vi "WiseDrive.vi"(8 "error in":errorcluster, 11 "Joystick Input":dbl(slide) scale=-1.0..1.0) -> (0 "error out":errorcluster, 3 "Throttle":dbl)   [LabVIEW 2015]
panel:
  in  "Low slope":dbl=0.5
  in  "Switch value":dbl=0.7
  # "remember to set as default to configure"
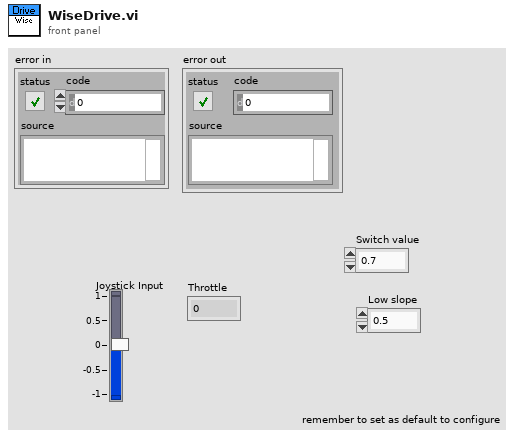
[diagram p1: front panel]
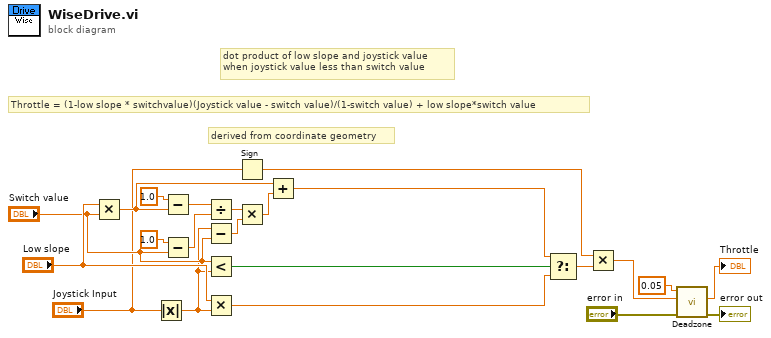
[diagram p0: block diagram]
diagram:
  # "derived from coordinate geometry"
  # "Throttle = (1-low slope * switchvalue)(Joystick value - switch value)/(1-switch value) + low slope*switch value"
  # "dot product of low slope and joystick value \nwhen joystick value less than switch value"
  n1 = Multiply(x="Low slope", y="Switch value") -> (x*y=w14:dbl)
  n2 = Absolute Value(x="Joystick Input") -> (abs(x)=w5:dbl)
  n3 = Subtract(x=1.0, y=w14) -> (x-y=w13:dbl)
  n4 = Subtract(x=1.0, y="Switch value") -> (x-y=w11:dbl)
  n5 = Divide(x=w13, y=w11) -> (x/y=w10:dbl)
  n6 = Subtract(x=w5, y="Switch value") -> (x-y=w9:dbl)
  n7 = Less?(x="Switch value", y=w5) -> (x < y?=w17:bool)
  n8 = Multiply(x="Low slope", y=w5) -> (x*y=w18:dbl)
  n9 = Sign(1:"Joystick Input") -> (0:w3:dbl)
  n10 = Multiply(x=w10, y=w9) -> (x*y=w8:dbl)
  n11 = Add(x=w14, y=w8) -> (x+y=w16:dbl)
  n12 = Select(t=w16, s=w17, f=w18) -> (s? t:f=w2:dbl)
  n13 = Multiply(x=w3, y=w2) -> (x*y=w1:dbl)
  n14 = call "Deadzone.vi"("error in"="error in", "Input"=w1, "Deadzone"=0.05) -> ("error out"=→"error out":errorcluster, "Output"=→"Throttle":dbl)  [unwired: 6 in, 1 out]
